vi "Manage User Presets.vi"(8 "error in (no error)":errorcluster, 9 "Load File (\"UserPreset.sta\")":string="UserPreset.sta", 10 "Action (0: Save)":i32(ring) items=["Save", "Load", "Perform"], 11 "VISA resource name":refnum<visa-resource-name>) -> (0 "error out":errorcluster, 3 "VISA resource name out":refnum<visa-resource-name>)   [LabVIEW 2018, in "Keysight PNA Series.lvlib"]
doc: "Loads, saves or performs a user preset."
uses:
  Keysight PNA Series.lvlib
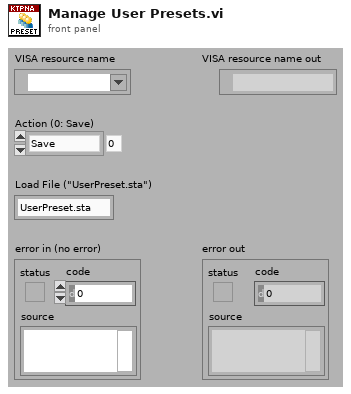
[diagram p1: front panel]
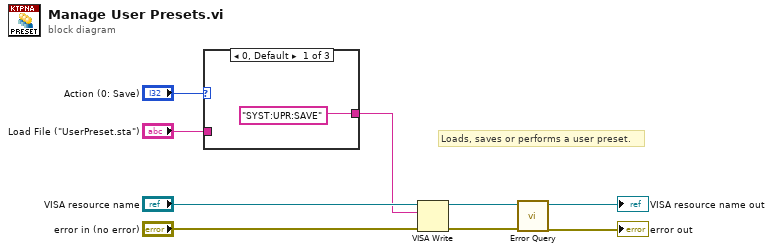
[diagram p0: block diagram]
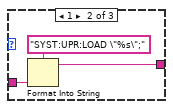
[diagram p2: hidden frame]
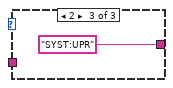
[diagram p3: hidden frame]
diagram:
  # "Loads, saves or performs a user preset."
  n1 = case shown="0, Default" "Action (0: Save)" {
    tunnel: ["SYST:UPR:SAVE" w11 "SYST:UPR"] -> w1
    tunnel: "Load File (\"UserPreset.sta\")" -> [_ w12 _]
    frame 0, Default {
    }
    frame 1 {
      n2 = Format Into String(format string="SYST:UPR:LOAD \"%s\";", w12) -> (resulting string=w11:string)  [unwired: 2 in, 1 out]
    }
    frame 2 {
    }
  }
  n3 = VISA Write(VISA resource name="VISA resource name", write buffer=w1, error in (no error)="error in (no error)") -> (VISA resource name out=w7:refnum<visa-resource-name>, error out=w6:errorcluster)  [unwired: 1 out]
  n4 = call "Error Query.vi"("error in (no error)"=w6, "VISA resource name"=w7) -> ("error out"=→"error out":errorcluster, "VISA resource name out"=→"VISA resource name out":refnum<visa-resource-name>)  [unwired: 6 in, 2 out]
